vi "Vision Processing.vi"() -> ()   [LabVIEW 2011]
doc: "This VI runs in parallel to other tasks. It gets images from the camera, processes them for color or shape and use that information to affect robot behavior."
uses:
  <vilib>/Rock Robotics/WPI/Camera/WPI_CameraWhite Balance Values.ctl
  Robot Global Data.vi
  <vilib>/vision/NI_Vision_Development_Module.lvlib
panel:
  in  "Turret Speed Limit":dbl=0.3
  out "Number of Rectangles Visible":dbl
  out "Y Position Array":dbl[](array[numeric])
  out "X Position Array":dbl[](array[numeric])
  out "Processed Image":T1(plugin-control)
  out "Original Image":T1(plugin-control)
  in  "Annotate":bool=TRUE
  in  "Particle Count Limit":i32=10
  in  "Area Size Limit":i32=444
  in  "Range":cluster{"Lower value":sgl, "Upper value":sgl}={"Lower value"=120.0, "Upper value"=255.0}
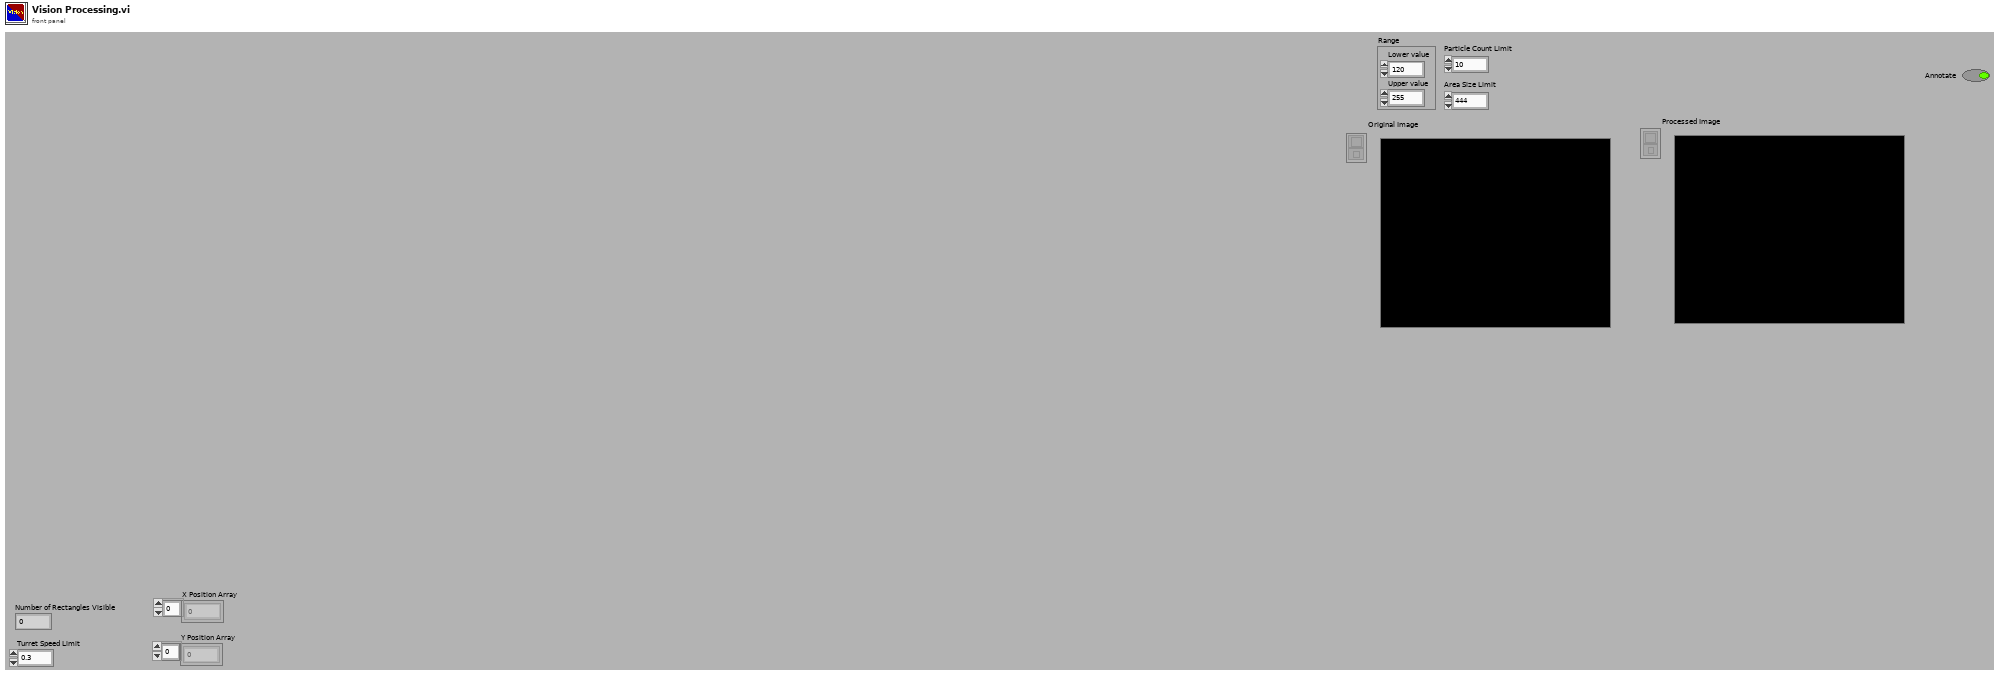
[diagram p1: front panel]
types:
  T1 = typedef "IMAQ Image.ctl" = refnum<image>
  T2 = cluster{"Rect Coverage":dbl, "Aspect Ratio":dbl, "X Edge Strength":dbl, "Y Edge Strength":dbl}
  T3 = cluster{"Position":cluster{"X":dbl, "Y":dbl}, "Distance (ft)":dbl}[]
  T4 = typedef "WPI_CameraWhite Balance Values.ctl" = enum16{"Auto", "Fixed indoor", "Fixed outdoor 1", "Fixed outdoor 2", "Fixed fluorescent 1", "Fixed fluorescent 2", "Hold current"}
  T5 = typedef "Image Type" = u32
  T6 = typedef "WPI_CameraImageSize.ctl" = enum16{"640x480", "320x240", "160x120"}
  T7 = cluster{"fps":i32, "compression":i32, "Image Size":T6}
  T8 = typedef "WPI_CameraDevRef.ctl" = cluster{"Camera Address":string, "CameraStatus":errorcluster, "Acquire Image Notifier":refnum<notifier>}
  T9 = cluster{cluster{"Left":dbl, "Top":dbl, "Right":dbl, "Bottom":dbl}, dbl[]}[]
  T10 = cluster{"Left":dbl, "Top":dbl, "Right":dbl, "Bottom":dbl}
  T11 = cluster{"Target Center (-1 to 1)":cluster{"X":dbl, "Y":dbl}, "Distance (ft)":dbl}
  T12 = cluster{"Target Center (-1 to 1)":cluster{"X":dbl, "Y":dbl}, "Distance (ft)":dbl}[]
  T13 = cluster{"Axis 1":dbl, "Axis 2":dbl, "Axis 3":dbl, "Axis 4":dbl, "Axis 5":dbl, "Axis 6":dbl, "Button 1":bool, "Button 2":bool, "Button 3":bool, "Button 4":bool, "Button 5":bool, "Button 6":bool, "Button 7":bool, "Button 8":bool, "Button 9":bool, "Button 10":bool, "Button 11":bool, "Button 12":bool}
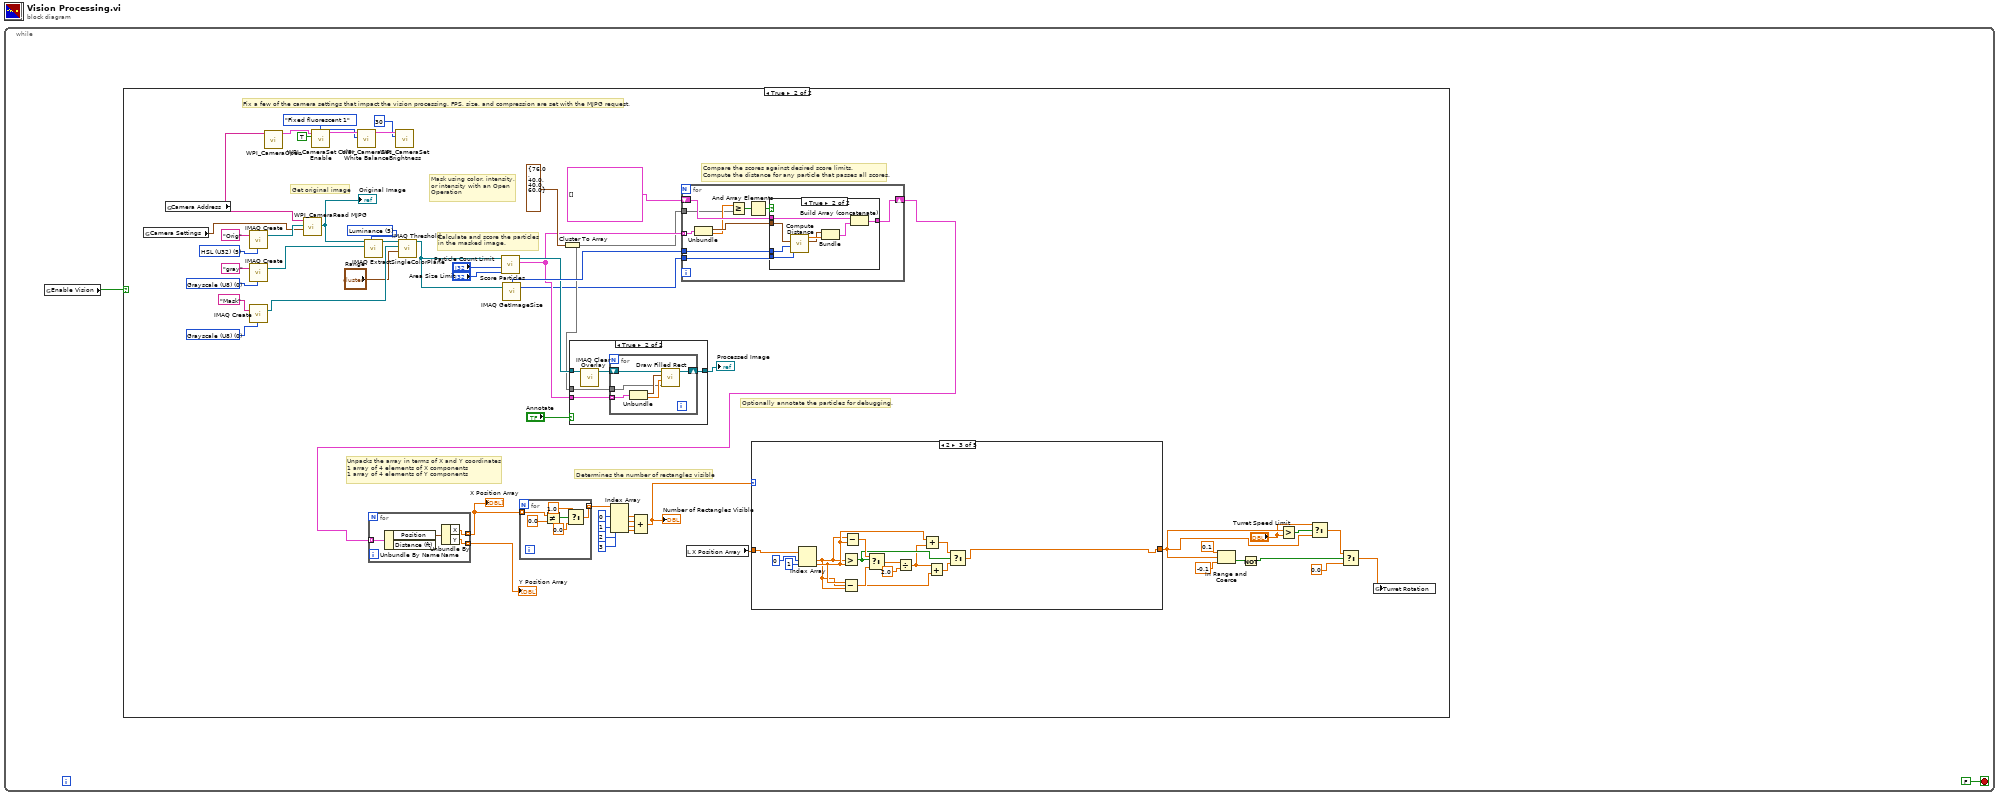
[diagram p0: block diagram]
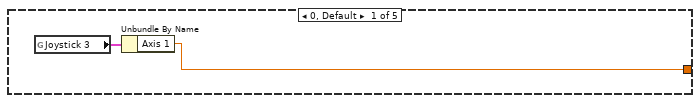
[diagram p3: hidden frame]
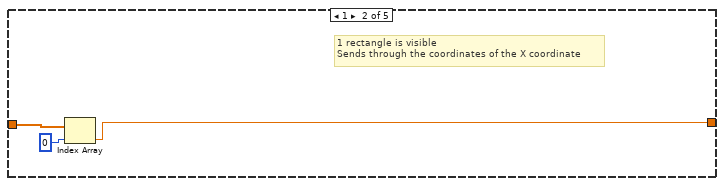
[diagram p4: hidden frame]
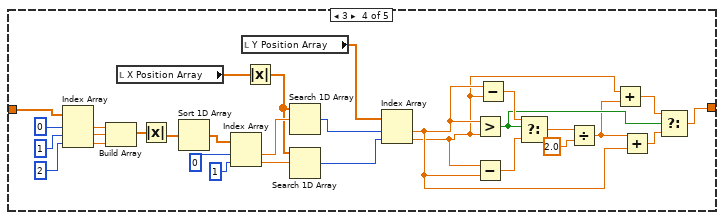
[diagram p5: hidden frame]
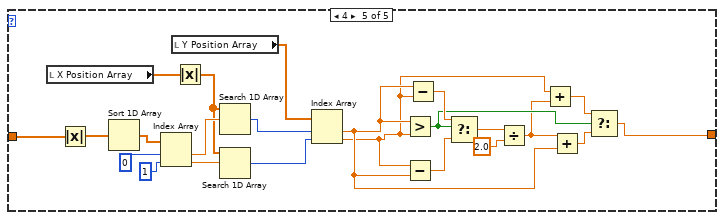
[diagram p6: hidden frame]
diagram:
  n1 = while {
    stop <- FALSE stop-if-true
    n2 = global read "Robot Global Data.vi" "Enable Vision"() -> (w1:bool)
    n3 = case shown="True" w1 {
      frame False {
      }
      frame True {
        w31 = 5 items=["Red", "Green", "Blue", "Hue", "Saturation", "Luminance", "Value", "Intensity"] ("Color Plane")
        w52 = T5 0 items=["Grayscale (U8)", "Grayscale (I16)", "Grayscale (SGL)", "Complex (CSG)", "RGB (U32)", "HSL (U32)", "RGB (U64)", "Grayscale (U16)"] ("Image Type")
        w56 = T5 5 items=["Grayscale (U8)", "Grayscale (I16)", "Grayscale (SGL)", "Complex (CSG)", "RGB (U32)", "HSL (U32)", "RGB (U64)", "Grayscale (U16)"] ("Image Type")
        w59 = T5 0 items=["Grayscale (U8)", "Grayscale (I16)", "Grayscale (SGL)", "Complex (CSG)", "RGB (U32)", "HSL (U32)", "RGB (U64)", "Grayscale (U16)"] ("Image Type")
        # "Determines the number of rectangles visible"
        # "Unpacks the array in terms of X and Y coordinates\n1 array of 4 elements of X components\n1 array of 4 elements of Y components"
        # "Optionally annotate the particles for debugging."
        # "Compare the scores against desired score limits.\nCompute the distance for any particle that passes all scores."
        # "Calculate and score the particles\nin the masked image."
        # "Mask using color, intensity,\nor intensity with an Open\nOperation"
        # "Get original image"
        # "Fix a few of the camera settings that impact the vision processing. FPS, size, and compression are set with the MJPG request."
        n4 = global read "Robot Global Data.vi" "Camera Settings"() -> (w43:T7)
        n5 = global read "Robot Global Data.vi" "Camera Address"() -> (w44:string)
        n6 = call "IMAQ Create"("Image Name"="Orig", "Image Type"=w56) -> ("New Image"=w55:T1)  [unwired: 2 in, 2 out]
        n7 = call "IMAQ Create"("Image Name"="gray", "Image Type"=w59) -> ("New Image"=w54:T1)  [unwired: 2 in, 2 out]
        n8 = call "IMAQ Create"("Image Name"="Mask", "Image Type"=w52) -> ("New Image"=w51:T1)  [unwired: 2 in, 2 out]
        n9 = call <vilib>:"WPI_CameraOpen.vi"("Camera Address"=w44) -> ("CameraDevRef"=w50:T8)  [unwired: 9 in, 1 out]
        n10 = call <vilib>:"WPI_CameraRead MJPG.vi"("Camera Settings"=w43, "Image"=w55, "address"=w44) -> ("Image Out"=w28:T1)  [unwired: 7 in, 1 out]
        "Original Image" <- w28
        n11 = call <vilib>:"WPI_CameraSet Color Enable.vi"("Color Enabled"=TRUE, "CameraDevRef"=w50) -> ("CameraDevRef Out"=w48:T8)  [unwired: 8 in, 1 out]
        n12 = call <vilib>:"WPI_CameraSet White Balance.vi"("White Balance"=WPI_CameraWhite_Balance_Values."Fixed fluorescent 1", "CameraDevRef"=w48) -> ("CameraDevRef Out"=w46:T8)  [unwired: 8 in, 1 out]
        n13 = call "IMAQ ExtractSingleColorPlane"("Color Plane"=w31, "Image Dst"=w54, "Image Src"=w28) -> ("Image Dst Out"=w29:T1)  [unwired: 1 in, 7 out]
        n14 = call <vilib>:"WPI_CameraSet Brightness.vi"("Brightness"=30, "CameraDevRef"=w46) -> ()  [unwired: 8 in, 2 out]
        n15 = call "IMAQ Threshold"("Range"="Range", "Image Dst"=w51, "Image Src"=w29) -> ("Image Dst Out"=w27:T1)  [unwired: 3 in, 5 out]
        n16 = call "Score Particles.vi"("Area Size Limit"="Area Size Limit", "Particle Count Limit"="Particle Count Limit", "Image Refnum in"=w27) -> ("Scored Particle Info"=w38:T9, "Image Refnum out"=w41:T1)  [unwired: 7 in]
        n17 = call "IMAQ GetImageSize"("Image"=w27) -> ("Y Resolution"=w32:i32, "X Resolution"=w42:i32)  [unwired: 3 in, 1 out]
        n18 = Cluster To Array(cluster=T2 {"Rect Coverage"=76.0, "Aspect Ratio"=40.0, "X Edge Strength"=40.0, "Y Edge Strength"=60.0} ("Score Limits")) -> (array=w36:dbl[])
        n19 = case shown="True" "Annotate" {
          tunnel: w41 -> [w142 w147]
          tunnel: [w142 w146] -> w39
          tunnel: w38 -> [_ w144]
          tunnel: w36 -> [_ w143]
          frame False {
          }
          frame True {
            n20 = call "IMAQ Clear Overlay"("Image"=w147) -> ("Image Out"=w145:T1)  [unwired: 2 in, 8 out]
            n21 = for {
              shift-right: [w152] -> w146
              shift-left: w145 -> [w153]
              tunnel: w144 -> [w149] mode=indexing
              tunnel: w143 -> [w148]
              n22 = Unbundle(w149) -> (w150:T10, w151:dbl[])
              n23 = call "Draw Filled Rect.vi"("Limits"=w148, "Scores"=w151, "Bounding Box"=w150, "image in"=w153) -> ("image out"=w152:T1)  [unwired: 7 in]
            }
          }
        }
        "Processed Image" <- w39
        n24 = for {
          shift-right: [w162] -> w4
          shift-left: T3 [] -> [w163]
          tunnel: w42 -> [w161]
          tunnel: w38 -> [w159] mode=indexing
          tunnel: w36 -> [w155]
          tunnel: w32 -> [w154]
          n25 = Unbundle(w159) -> (w160:T10, w156:dbl[])
          n26 = Greater Or Equal?(x=w156, y=w155) -> (x >= y?=w158:bool[])
          n27 = And Array Elements(Boolean array=w158) -> (logical AND=w157:bool)
          n28 = case shown="True" w157 {
            tunnel: w163 -> [w164 w172]
            tunnel: [w164 w171] -> w162
            tunnel: w160 -> [_ w167]
            tunnel: w161 -> [_ w169]
            tunnel: w154 -> [_ w165]
            frame False {
            }
            frame True {
              n29 = call "Compute Distance.vi"("Y Image Resolution"=w165, "X Image Resolution"=w169, "Bounding Box"=w167) -> ("Target Center (-1 to 1)"=w166:cluster{"X":dbl, "Y":dbl}, "Distance (ft)"=w168:dbl)  [unwired: 7 in]
              n30 = Bundle("Target Center (-1 to 1)"=w166, "Distance (ft)"=w168) -> (w170:T11)  [unwired: 1 in]
              n31 = Build Array (concatenate)(w172, w170) -> (w171:T12)
            }
          }
        }
        n32 = for {
          tunnel: [w140] -> w5 mode=indexing
          tunnel: [w139] -> w17 mode=indexing
          tunnel: w4 -> [w138] mode=indexing
          n33 = Unbundle By Name(w138) -> ("Position"=w141:cluster{"X":dbl, "Y":dbl})  [unwired: 1 out]
          n34 = Unbundle By Name(w141) -> ("X"=w139:dbl, "Y"=w140:dbl)
        }
        "X Position Array" <- w17
        "Y Position Array" <- w5
        n35 = for {
          tunnel: w17 -> [w64] mode=indexing
          tunnel: [w60] -> w18 mode=indexing
          n36 = Not Equal?(x=w64, y=0.0) -> (x != y?=w63:bool)
          n37 = Select(t=1.0, s=w63, f=0.0) -> (s? t:f=w60:dbl)
        }
        n38 = Index Array(array=w18, index #1=0 ("index"), index #2=1 ("index"), index #3=2 ("index"), index #4=3 ("index")) -> (element #1=w20:dbl, element #2=w19:dbl, element #3=w21:dbl, element #4=w22:dbl)
        n39 = Compound Arithmetic op=ADD(w20, w19, w21, w22) -> (w3:dbl)
        "Number of Rectangles Visible" <- w3
        n40 = local read "X Position Array"() -> (w6:dbl[])
        n41 = case shown="2" w3 {
          tunnel: w6 -> [_ w70 w72 w86 w116]
          tunnel: [w66 w68 w71 w85 w115] -> w16
          frame 0, Default {
            n42 = global read "Robot Global Data.vi" "Joystick 3"() -> (w67:T13)
            n43 = Unbundle By Name(w67) -> ("Axis 1"=w66:dbl)
          }
          frame 1 {
            # "1 rectangle is visible\nSends through the coordinates of the X coordinate"
            n44 = Index Array(array=w70, index=0) -> (element=w68:dbl)
          }
          frame 2 {
            n45 = Index Array(array=w72, index #1=0 ("index"), index #2=1 ("index")) -> (element #1=w73:dbl, element #2=w74:dbl)
            n46 = Greater?(x=w73, y=w74) -> (0:w78:bool)
            n47 = Subtract(x=w74, y=w73) -> (x-y=w81:dbl)
            n48 = Subtract(x=w73, y=w74) -> (x-y=w82:dbl)
            n49 = Select(t=w82, s=w78, f=w81) -> (s? t:f=w80:dbl)
            n50 = Divide(x=w80, y=2.0) -> (x/y=w75:dbl)
            n51 = Add(x=w74, y=w75) -> (x+y=w77:dbl)
            n52 = Add(x=w75, y=w73) -> (x+y=w76:dbl)
            n53 = Select(t=w77, s=w78, f=w76) -> (s? t:f=w71:dbl)
          }
          frame 3 {
            n54 = Index Array(array=w86, index #1=0 ("index"), index #2=1 ("index"), index #3=2 ("index")) -> (element #1=w111:dbl, element #2=w110:dbl, element #3=w109:dbl)
            n55 = Build Array(w111, w110, w109) -> (w108:dbl[])
            n56 = local read "X Position Array"() -> (w101:dbl[])
            n57 = Absolute Value(x=w108) -> (abs(x)=w107:dbl[])
            n58 = Sort 1D Array(array=w107) -> (sorted array=w106:dbl[])
            n59 = Index Array(array=w106, index #1=0 ("index"), index #2=1 ("index")) -> (element #1=w103:dbl, element #2=w102:dbl)
            n60 = local read "Y Position Array"() -> (w99:dbl[])
            n61 = Absolute Value(x=w101) -> (abs(x)=w87:dbl[])
            n62 = Search 1D Array(1D array=w87, element=w103) -> (index of element=w100:i32)  [unwired: 1 in]
            n63 = Search 1D Array(1D array=w87, element=w102) -> (index of element=w98:i32)  [unwired: 1 in]
            n64 = Index Array(array=w99, index #1=w100, index #2=w98) -> (element #1=w89:dbl, element #2=w88:dbl)
            n65 = Greater?(x=w89, y=w88) -> (0:w93:bool)
            n66 = Subtract(x=w88, y=w89) -> (x-y=w96:dbl)
            n67 = Subtract(x=w89, y=w88) -> (x-y=w97:dbl)
            n68 = Select(t=w97, s=w93, f=w96) -> (s? t:f=w95:dbl)
            n69 = Divide(x=w95, y=2.0) -> (x/y=w90:dbl)
            n70 = Add(x=w88, y=w90) -> (x+y=w92:dbl)
            n71 = Add(x=w90, y=w89) -> (x+y=w91:dbl)
            n72 = Select(t=w92, s=w93, f=w91) -> (s? t:f=w85:dbl)
          }
          frame 4 {
            n73 = local read "X Position Array"() -> (w131:dbl[])
            n74 = Absolute Value(x=w116) -> (abs(x)=w137:dbl[])
            n75 = Sort 1D Array(array=w137) -> (sorted array=w136:dbl[])
            n76 = Index Array(array=w136, index #1=0 ("index"), index #2=1 ("index")) -> (element #1=w133:dbl, element #2=w132:dbl)
            n77 = local read "Y Position Array"() -> (w129:dbl[])
            n78 = Absolute Value(x=w131) -> (abs(x)=w117:dbl[])
            n79 = Search 1D Array(1D array=w117, element=w133) -> (index of element=w130:i32)  [unwired: 1 in]
            n80 = Search 1D Array(1D array=w117, element=w132) -> (index of element=w128:i32)  [unwired: 1 in]
            n81 = Index Array(array=w129, index #1=w130, index #2=w128) -> (element #1=w119:dbl, element #2=w118:dbl)
            n82 = Greater?(x=w119, y=w118) -> (0:w123:bool)
            n83 = Subtract(x=w118, y=w119) -> (x-y=w126:dbl)
            n84 = Subtract(x=w119, y=w118) -> (x-y=w127:dbl)
            n85 = Select(t=w127, s=w123, f=w126) -> (s? t:f=w125:dbl)
            n86 = Divide(x=w125, y=2.0) -> (x/y=w120:dbl)
            n87 = Add(x=w118, y=w120) -> (x+y=w122:dbl)
            n88 = Add(x=w120, y=w119) -> (x+y=w121:dbl)
            n89 = Select(t=w122, s=w123, f=w121) -> (s? t:f=w115:dbl)
          }
        }
        n90 = In Range and Coerce(upper limit=0.1, x=w16, lower limit=-0.1) -> (In Range?=w12:bool)  [unwired: 1 out]
        n91 = Not(x=w12) -> (.not. x?=w11:bool)
        n92 = Greater?(x=w16, y="Turret Speed Limit") -> (0:w9:bool)
        n93 = Select(t="Turret Speed Limit", s=w9, f=w16) -> (s? t:f=w7:dbl)
        n94 = Select(t=w7, s=w11, f=0.0) -> (s? t:f=w15:dbl)
        n95 = global write "Robot Global Data.vi" "Turret Rotation"(w15) -> ()
      }
    }
  }
